vi "Find GlobalStat Value.vi"(3 "Array":u32[](array[numeric])) -> (1 "GlobalStat value":dbl)   [LabVIEW 2020, in "AIM ARINC 664 Engine.lvlib" / "Implementation.lvlib" / "Monitor Execution Unit.lvclass"]
uses:
  Monitor Execution Unit.lvclass
  Monitor Execution Unit.lvclass/Monitor Execution Unit.ctl
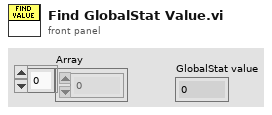
[diagram p1: front panel]
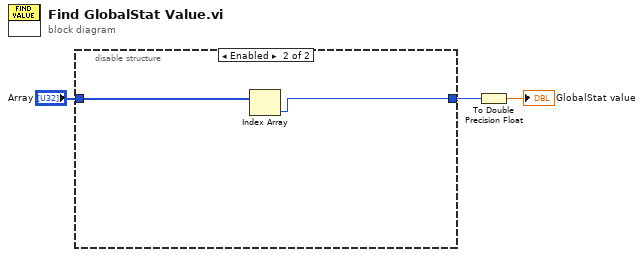
[diagram p0: block diagram]
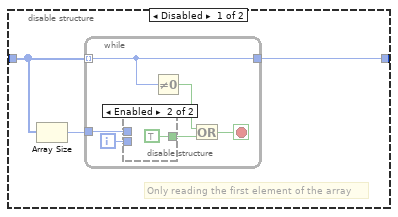
[diagram p2: hidden frame]
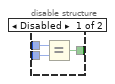
[diagram p3: hidden frame]
diagram:
  n1 = disable-structure shown="Enabled" {
    disable-tunnel: [w6 w17] -> w3
    disable-tunnel: "Array" -> [w5 w18]
    frame Disabled {
      # "Only reading the first element of the array"
      n2 = Array Size(array=w5) -> (size(s)=w4:i32)
      n3 = while {
        tunnel: w5 -> [w12] mode=indexing
        tunnel: [w12] -> w6
        tunnel: w4 -> [w8]
        i -> [w9]
        stop <- w10 stop-if-true
        n4 = disable-structure shown="Enabled" {
          disable-tunnel: w9 -> [w15 _]
          disable-tunnel: w8 -> [w14 _]
          disable-tunnel: [w13 TRUE] -> w7
          frame Disabled {
            n5 = Equal?(x=w14, y=w15) -> (x = y?=w13:bool)
          }
          frame Enabled {
          }
        }
        n6 = Not Equal To 0?(x=w12) -> (x != 0?=w11:bool)
        n7 = Or(x=w11, y=w7) -> (x .or. y?=w10:bool)
      }
    }
    frame Enabled {
      n8 = Index Array(array=w18) -> (element=w17:u32)  [unwired: 1 in]
    }
  }
  n9 = To Double Precision Float(number=w3) -> (double precision float=→"GlobalStat value":dbl)
